vi "RunSelfCheck5.vi"(1 "Select_CalPwrMeters":bool=TRUE, 2 "Select_SplitterPwr":bool=TRUE, 3 "error in (no error)":errorcluster, 4 "Select_Processor_HV_Flag":bool=TRUE, 5 "File name base":string="SelfCheck5_") -> (0 "error out":errorcluster)   [LabVIEW 2009]
doc: "Measures a collection of system calibration variables, growing awith time, a work in progress."
uses:
  Rvp8PowerData.ctl
panel:
  in  "startGateTestPulse":i32=970
  in  "nGates TestPulse":i32=10
  in  "nSamplesTestPulse":i32=1000
  out "RVP8_testPulse_measurement":T1 {"time" format="%<%H:%M:%S\n%Y/%m/%d>T"}
  in  "SG Freq GHz 2":dbl=2.795 format="%#.5f"
  out "SelfCheckEndTime":timestamp
  out "SelfCheckStartTime":timestamp
  out "OutputFileName":string
  out "or Tee, Confirm That Pol Sw 7222 = 0 = SCPI closed = local control Tee, Confirm That Pol Sw 7222 = 1 = SCPI open for processor 2":i32
  out "For Tee, Confirm That Pol Sw 7223 = 0 =  SCPI closed \"honly\" 2":i32
  out "or Tee, Confirm That Pol Sw 7222 = 0 = SCPI closed = local control Tee, Confirm That Pol Sw 7222 = 1 = SCPI open for processor":i32
  out "For Tee, Confirm That Pol Sw 7223 = 0 =  SCPI closed \"honly\"":i32
  out "RVP8_Noise_Injection_NoAmp_Normal":T1 {"time" format="%<%H:%M:%S\n%Y/%m/%d>T"}
  out "RVP8_SigGen_NoAmp_Normal":T1 {"time" format="%<%H:%M:%S\n%Y/%m/%d>T"}
  out "dBAvg Power Meter Noise Floor (dBm)":dbl format="%#.5f"
  in  "startGate burst RVP8":i32=-1
  in  "nGates burst RVP8":i32=1
  in  "nSamples burst RVP8":i32=1000
  out "RVP8 TxBurstHc":dbl
  out "RVP8_burstPulse_measurement":T1 {"time" format="%<%H:%M:%S\n%Y/%m/%d>T"}
  out "String_WgSw_Positions":string
  out "Initial Check  of Transmit Detector: TxUp=0 if not transmitting":i32
  out "RVP8_HighSigGen_Injection_Reversed":T1 {"time" format="%<%H:%M:%S\n%Y/%m/%d>T"}
  out "RVP8_HighSigGen_Injection_Normal":T1 {"time" format="%<%H:%M:%S\n%Y/%m/%d>T"}
  out "Updating Data File Time":string
  out "StringOfRelayCycles":string
  out "SSD TOF Tx Pwr Reading dB":dbl format="%#.6g"
  out "TOF Tx Pwr Reading dBm":dbl format="%#.6g"
  out "dB SSD SigGen Power NO Amp to splitter (dB)":dbl format="%.5f"
  out "dBAvg SigGen Power NO Amp to splitter (dBm)":dbl format="%.3f"
  out "dB SSD Inside Noise Box Power thru Amp to splitter (dB)":dbl format="%.5f"
  out "dBSSD SigGen Power thru Amp to splitter (dB)":dbl format="%.5f"
  out "RVP8_LowSigGen_Injection_Normal":T1 {"time" format="%<%H:%M:%S\n%Y/%m/%d>T"}
  out "RVP8_LowSigGen_Injection_Reversed":T1 {"time" format="%<%H:%M:%S\n%Y/%m/%d>T"}
  out "StartFracDaysSince01Jan1904":dbl format="%#.6g"
  in  "File name exten":string="csv"
  out "TxDetector Voltage":dbl
  out "Temp Inside Noise Box":dbl
  out "Temp Outside Noise Box":dbl
  out "RVP8_Noise_Injection_Reversed":T1 {"time" format="%<%H:%M:%S\n%Y/%m/%d>T"}
  out "RVP8_Noise_Injection_Normal":T1 {"time" format="%<%H:%M:%S\n%Y/%m/%d>T"}
  out "RVP8_outside_noise_box_normal":T1 {"time" format="%<%H:%M:%S\n%Y/%m/%d>T"}
  out "First RVP8 Time":dbl format="%#_9g"
  out "RVP8_background_noise_normal":T1 {"time" format="%<%H:%M:%S\n%Y/%m/%d>T"}
  out "+15V PS Voltage":dbl
  out "+24V PS Voltage":dbl
  out "Temp 34921T":dbl
  out "Temp TOF Pwr Sensor":dbl
  out "Temp Klystron":dbl
  out "Temp DL V":dbl
  out "Temp DL H":dbl
  out "Temp Circ V":dbl
  out "Temp Circ H":dbl
  out "Temp Outside":dbl
  out "Temp Delay":dbl
  out "dBAvg Inside Noise Box Power Thru Amp to splitter (dBm)":dbl format="%.3f"
  out "Temp Amp":dbl
  out "Temp Inside":dbl
  out "Temp Siggen":dbl
  out "Temp IFD":dbl
  out "First RVP8 azimuth":dbl
  out "First RVP8 elevation":dbl
  out "Temp LNA  V":dbl
  out "Temp LNA H":dbl
  out "Temp Pwr Sensor":dbl
  out "dBAvg SigGen Power thru Amp to splitter (dBm)":dbl format="%.3f"
  in  "Cal data directory":string="/home/operator/data"
  # "RECEIVER AND TEST EQUIPMENT SELF CHECKS & LOGGING VERSION #5:"
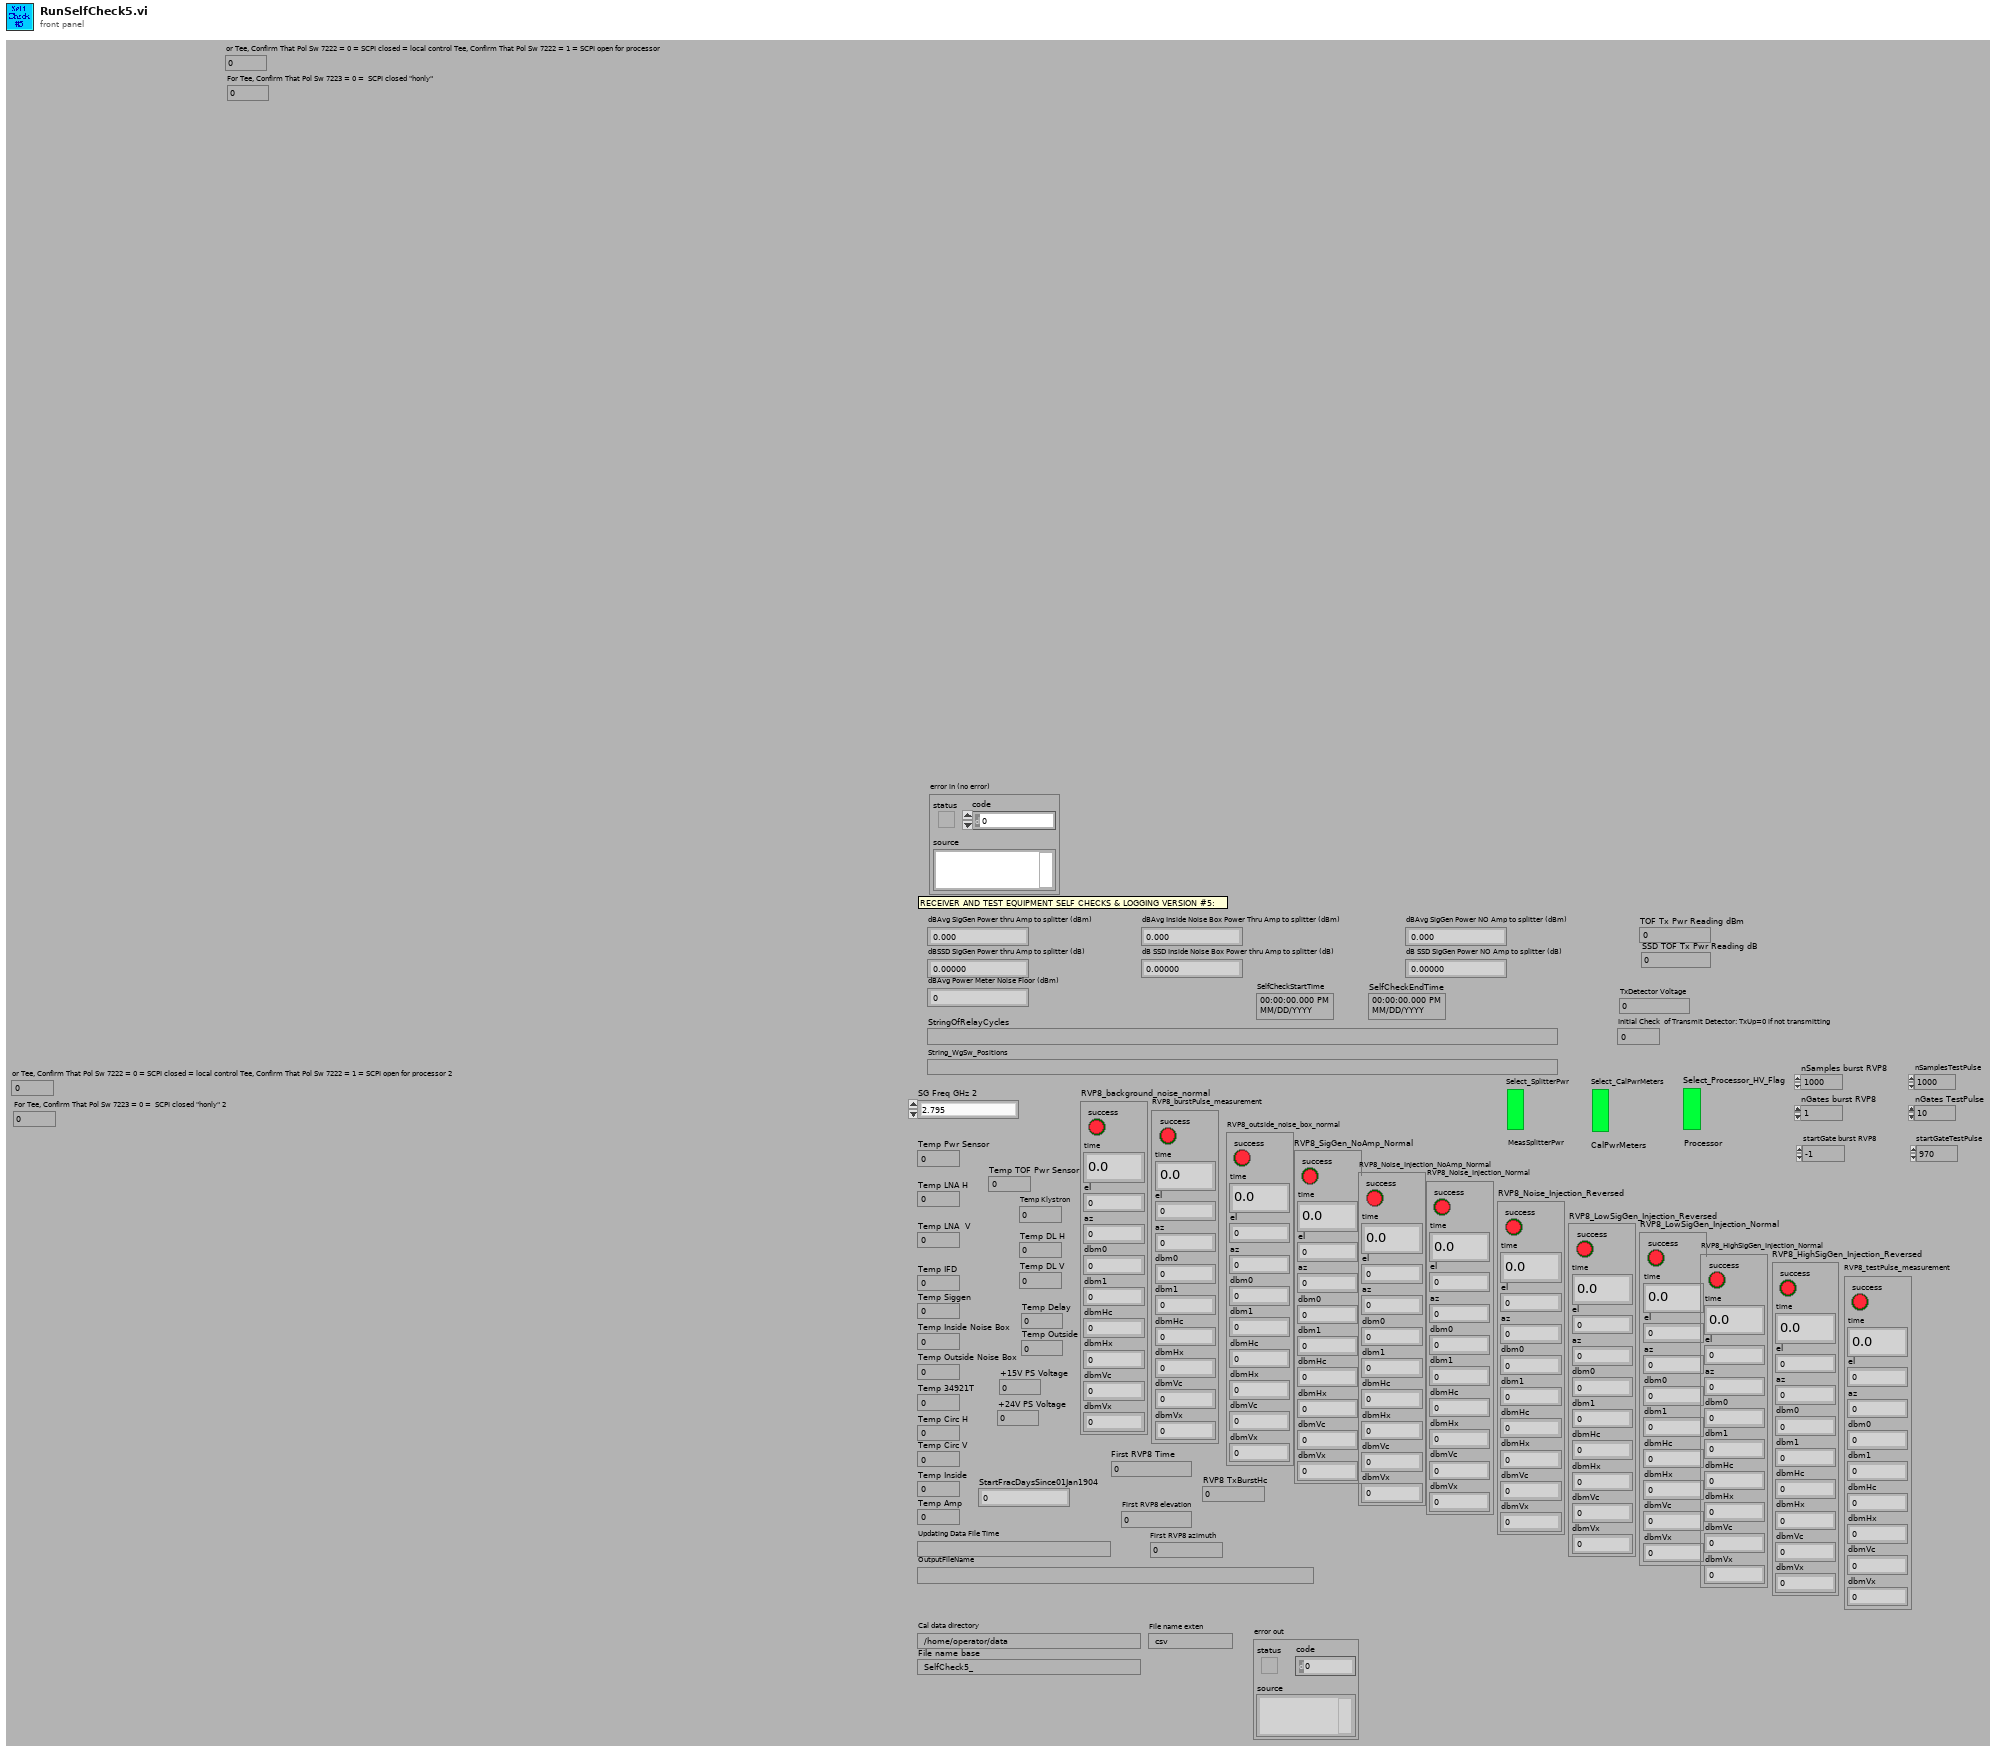
[diagram p1: front panel]
types:
  T1 = typedef "Rvp8PowerData.ctl" = cluster{"success":bool, "time":dbl, "el":dbl, "az":dbl, "dbm0":dbl, "dbm1":dbl, "dbmHc":dbl, "dbmHx":dbl, "dbmVc":dbl, "dbmVx":dbl}
  T2 = enum16{"open", "replace", "create", "open or create", "replace or create", "replace or create with confirmation"}
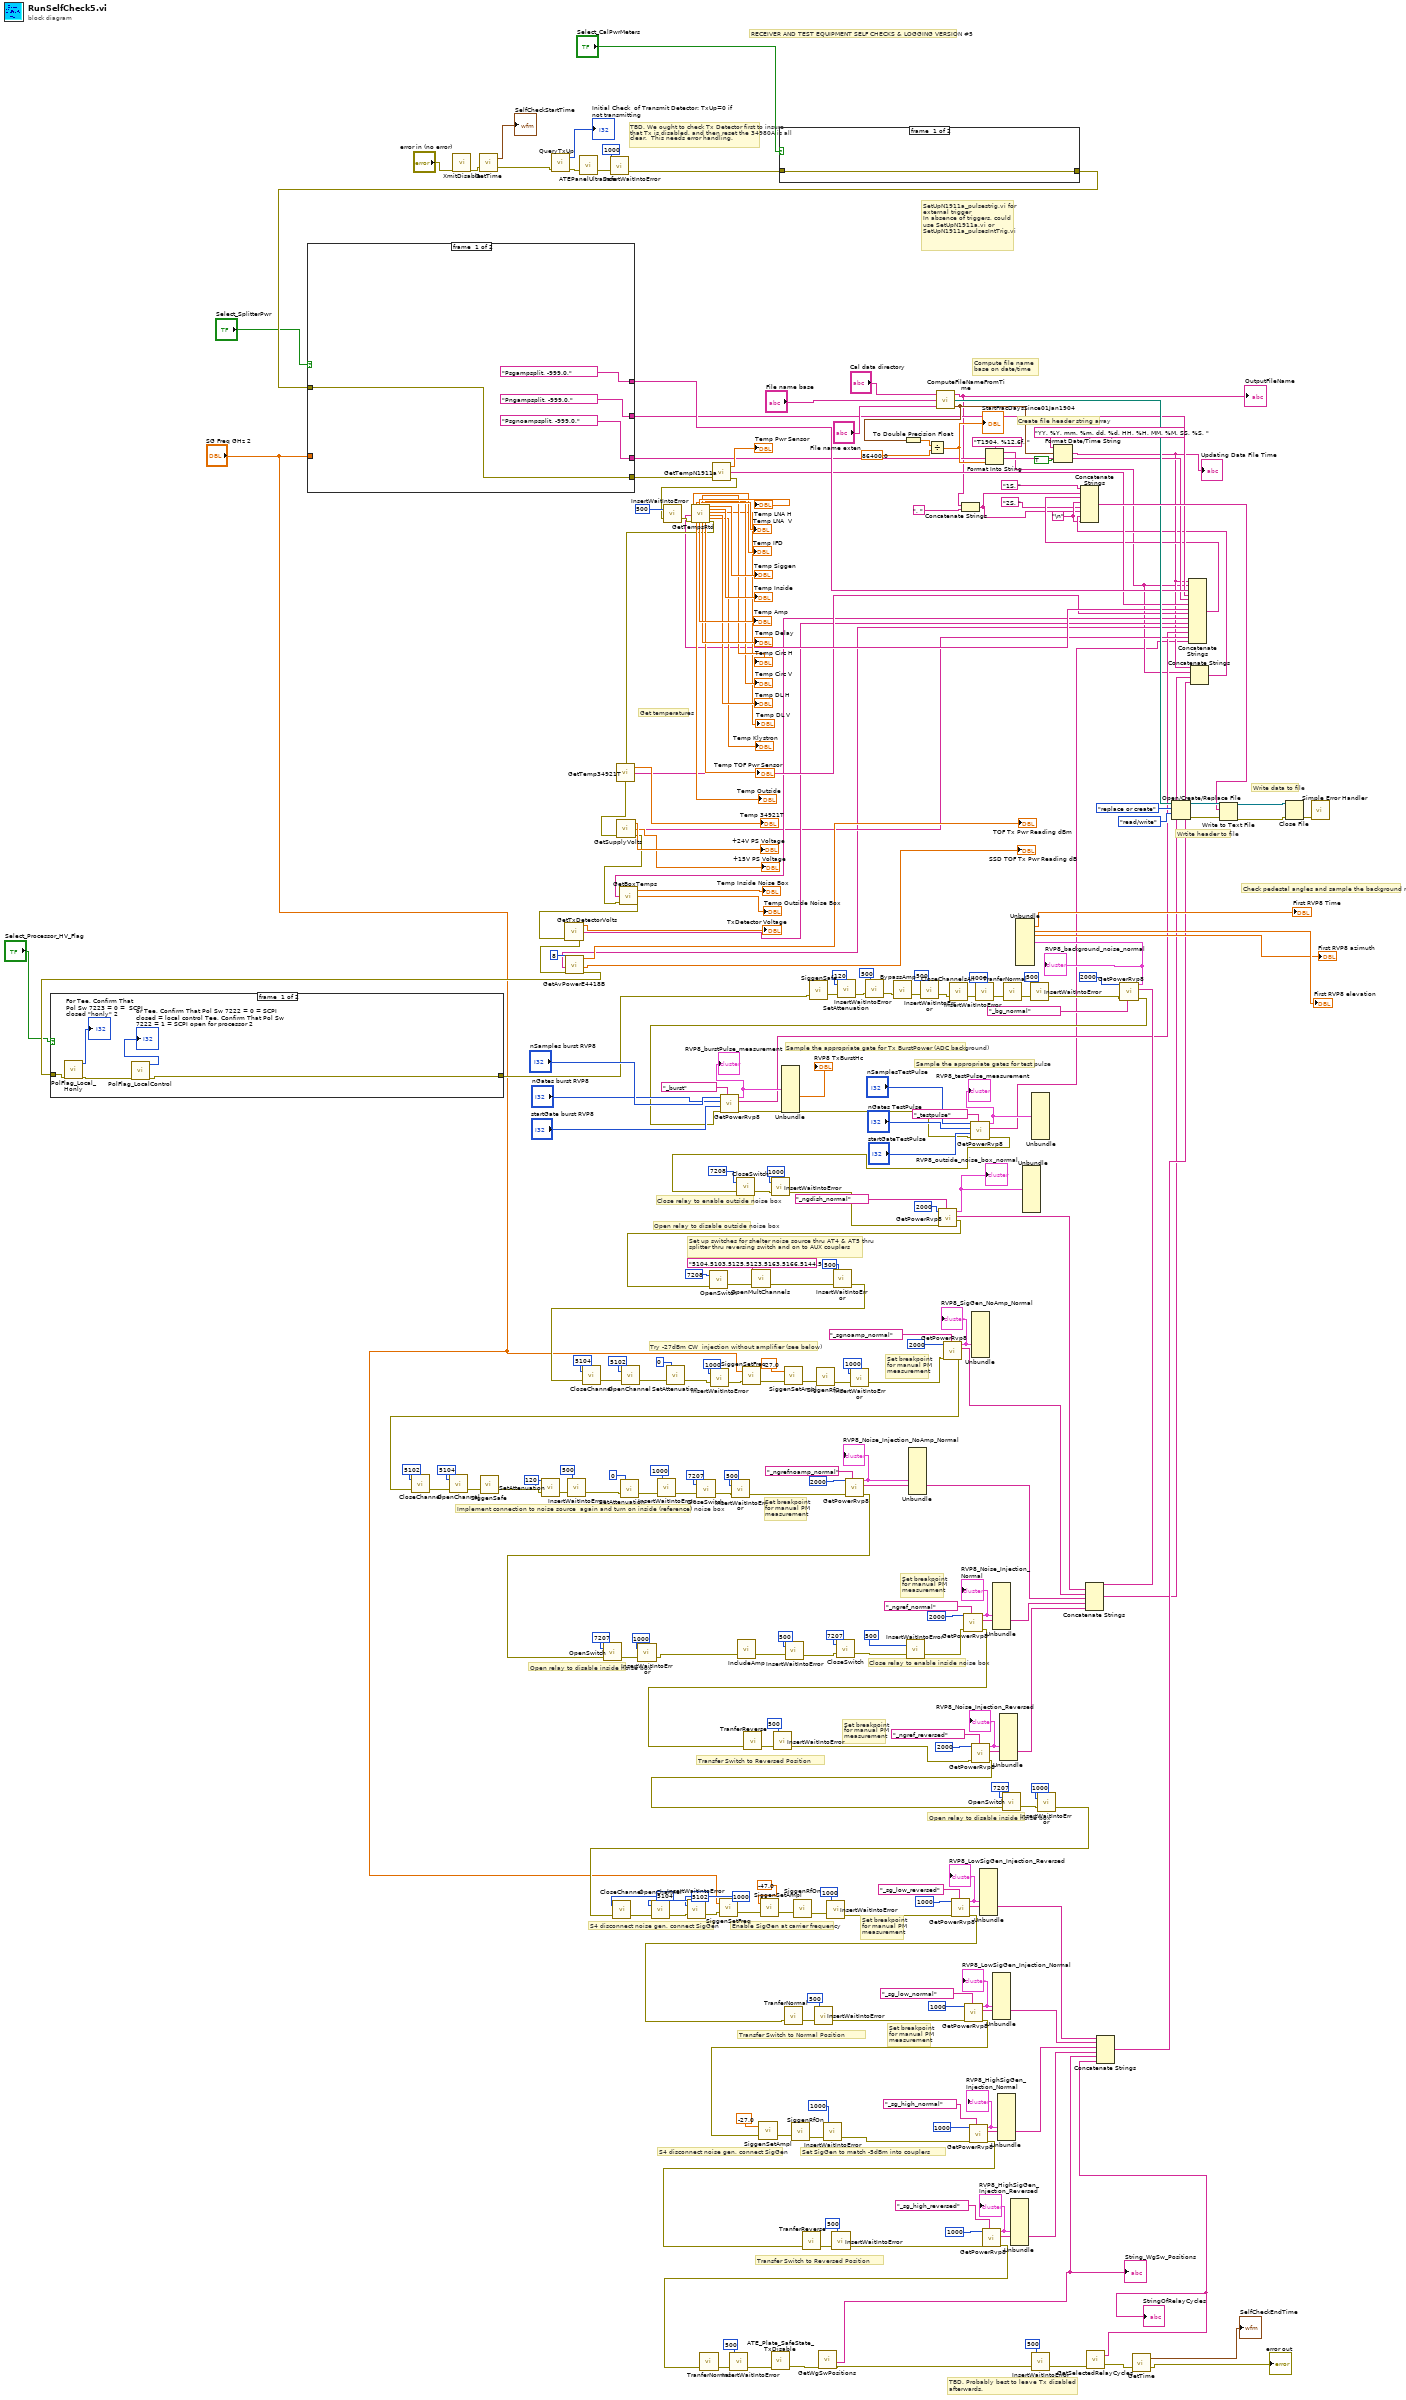
[diagram p0: block diagram]
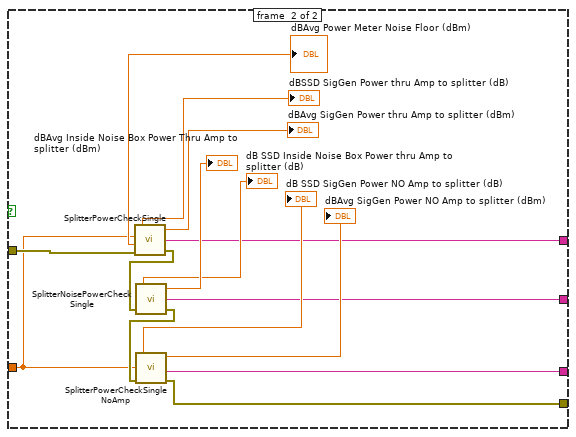
[diagram p2: hidden frame]
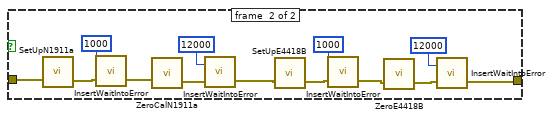
[diagram p3: hidden frame]
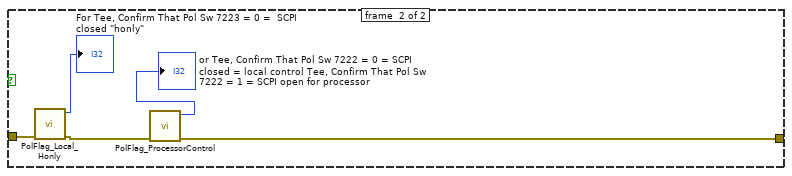
[diagram p4: hidden frame]
diagram:
  w80 = "\n"
  # "Sample the appropriate gates for test pulse"
  # "Set breakpoint for manual PM measurement"
  # "Set breakpoint for manual PM measurement"
  # "Set breakpoint for manual PM measurement"
  # "Set breakpoint for manual PM measurement"
  # "Set breakpoint for manual PM measurement"
  # "Set breakpoint for manual PM measurement"
  # "Open relay to disable inside noise box"
  # "Try -27dBm CW  injection without amplifier (see below)"
  # "Implement connection to noise source  again and turn on inside (reference) noise box"
  # "SetUpN1911a_pulsestrig.vi for external trigger\nIn absence of triggers, could use SetUpN1911a.vi or SetUpN1911a_pulsesIntTrig.vi"
  # "Sample the appropriate gate for Tx BurstPower (ADC background)"
  # "S4 disconnect noise gen, connect SigGen"
  # "Set SigGen to match -5dBm into couplers"
  # "Transfer Switch to Reversed Position"
  # "TBD. Probably best to leave Tx disabled afterwards."
  # "TBD. We ought to check Tx Detector first to insure that Tx is disabled, and then reset the 34980A is all clear.  This needs error handling."
  # "S4 disconnect noise gen, connect SigGen"
  # "Enable SigGen at carrier frequency"
  # "Transfer Switch to Normal Position"
  # "Transfer Switch to Reversed Position"
  # "Open relay to disable inside noise box"
  # "RECEIVER AND TEST EQUIPMENT SELF CHECKS & LOGGING VERSION #5"
  # "Close relay to enable inside noise box"
  # "Open relay to disable outside noise box"
  # "Close relay to enable outside noise box"
  # "Check pedestal angles and sample the background noise"
  # "Get temperatures"
  # "Write data to file"
  # "Wrtite header to file"
  # "Create file header string array"
  # "Set up switches for shelter noise source thru AT4 & AT5 thru splitter thru reversing switch and on to AUX couplers"
  # "Compute file name base on date/time"
  n1 = call "XmitDisable.vi"("error in (no error)"="error in (no error)") -> ("error out"=w15:errorcluster)  [unwired: 1 in, 5 out]
  n2 = call "GetTime.vi"("error in (no error)"=w15) -> ("error out"=w14:errorcluster, "CurrentTime"=→"SelfCheckStartTime":timestamp)  [unwired: 1 in]
  n3 = call "QueryTxUp.vi"("error in (no error)"=w14) -> ("error out"=w133:errorcluster, "IfTransmittingOne"=→"Initial Check  of Transmit Detector: TxUp=0 if not transmitting":i32)  [unwired: 1 in, 2 out]
  n4 = call "ATEPanelUltraSafe.vi"("error in (no error)"=w133) -> ("Error out"=w97:errorcluster)  [unwired: 2 in]
  n5 = call "InsertWaitIntoError.vi"("error in (no error)"=w97, "Wait (msecs)"=1000) -> ("error out"=w189:errorcluster)  [unwired: 1 in]
  n6 = case shown="True" "Select_CalPwrMeters" {
    tunnel: w189 -> [w267 w275]
    tunnel: [w267 w268] -> w154
    frame #0 {
    }
    frame #1 {
      n7 = call "SetUpN1911a.vi"("error in (no error)"=w275) -> ("error out"=w278:errorcluster)  [unwired: 2 in]
      n8 = call "InsertWaitIntoError.vi"("error in (no error)"=w278, "Wait (msecs)"=1000) -> ("error out"=w277:errorcluster)  [unwired: 1 in]
      n9 = call "ZeroCalN1911a.vi"("error in (no error)"=w277) -> ("error out"=w276:errorcluster)  [unwired: 2 in]
      n10 = call "InsertWaitIntoError.vi"("error in (no error)"=w276, "Wait (msecs)"=12000) -> ("error out"=w269:errorcluster)  [unwired: 1 in]
      n11 = call "SetUpE4418B.vi"("error in (no error)"=w269) -> ("error out"=w272:errorcluster)  [unwired: 2 in]
      n12 = call "InsertWaitIntoError.vi"("error in (no error)"=w272, "Wait (msecs)"=1000) -> ("error out"=w271:errorcluster)  [unwired: 1 in]
      n13 = call "ZeroE4418B.vi"("error in (no error)"=w271) -> ("error out"=w270:errorcluster)  [unwired: 2 in]
      n14 = call "InsertWaitIntoError.vi"("error in (no error)"=w270, "Wait (msecs)"=12000) -> ("error out"=w268:errorcluster)  [unwired: 1 in]
    }
  }
  n15 = case shown="True" "Select_SplitterPwr" {
    tunnel: [w284 w296] -> w155
    tunnel: w154 -> [w284 w290]
    tunnel: ["Psgampsplit, -999.0," w289] -> w118
    tunnel: ["Pngampsplit, -999.0," w288] -> w117
    tunnel: ["Psgnoampsplit, -999.0," w287] -> w116
    tunnel: "SG Freq GHz 2" -> [_ w285]
    frame #0 {
    }
    frame #1 {
      n16 = call "SplitterPowerCheckSingle.vi"("error in (no error)"=w290, "Select SG Freq GHz"=w285) -> ("error out"=w298:errorcluster, "String_PSG_Amp_Split"=w289:string, "dBAvg SigGen Power to splitter (dBm)"=→"dBAvg SigGen Power thru Amp to splitter (dBm)":dbl, "dBAvg Power Meter Noise Floor (dBm)"=→"dBAvg Power Meter Noise Floor (dBm)":dbl, "dBSSD SigGen Power to splitter (dB)"=→"dBSSD SigGen Power thru Amp to splitter (dB)":dbl)
      n17 = call "SplitterNoisePowerCheckSingle.vi"("error in (no error)"=w298) -> ("error out"=w295:errorcluster, "String_PNG_Amp_Split"=w288:string, "dBAvg Noise Power to splitter (dBm)"=→"dBAvg Inside Noise Box Power Thru Amp to splitter (dBm)":dbl, "dBSSD Noise Power to splitter (dB)"=→"dB SSD Inside Noise Box Power thru Amp to splitter (dB)":dbl)  [unwired: 1 in]
      n18 = call "SplitterPowerCheckSingleNoAmp.vi"("error in (no error)"=w295, "Select SG Freq GHz"=w285) -> ("error out"=w296:errorcluster, "String_PSG_Noamp_Split"=w287:string, "dBAvg SigGen Power to splitter (dBm)"=→"dBAvg SigGen Power NO Amp to splitter (dBm)":dbl, "dBSSD SigGen Power to splitter (dB)"=→"dB SSD SigGen Power NO Amp to splitter (dB)":dbl)  [unwired: 1 in, 1 out]
    }
  }
  n19 = call "GetTempN1911a.vi"("error in (no error)"=w155) -> ("Error out"=w250:errorcluster, "String_Temp_n1911a"=w115:string, "N1911a Temp (C)"=→"Temp Pwr Sensor":dbl)  [unwired: 2 in]
  n20 = call "InsertWaitIntoError.vi"("error in (no error)"=w250, "Wait (msecs)"=500) -> ("error out"=w252:errorcluster)  [unwired: 1 in]
  n21 = call "GetTempsRtd.vi"("error in (no error)"=w252) -> ("Temp IFD"=→"Temp IFD":dbl, "String_Temperatures"=w114:string, "Temp VLNA"=→"Temp LNA  V":dbl, "Temp Outside"=→"Temp Outside":dbl, "Temp HLNA"=→"Temp LNA H":dbl, "Temp ATE Amp"=→"Temp Amp":dbl, "Temp H Circ"=→"Temp Circ H":dbl, "Temp ATE delay"=→"Temp Delay":dbl, "Temp V Circ"=→"Temp Circ V":dbl, "Temp TOF Pwr"=→"Temp TOF Pwr Sensor":dbl, "Temp Siggen"=→"Temp Siggen":dbl, "Temp Inside"=→"Temp Inside":dbl, "Temp V Dummy"=→"Temp DL V":dbl, "Temp H Dummy"=→"Temp DL H":dbl, "Temp Klystron"=→"Temp Klystron":dbl, "error out"=w232:errorcluster)  [unwired: 2 in, 1 out]
  n22 = call "GetTemp34921T.vi"("error in (no error)"=w232) -> ("Error out"=w233:errorcluster, "String_Temp_34921T"=w113:string, "34921A Temp (C)"=→"Temp 34921T":dbl)  [unwired: 2 in]
  n23 = call "GetSupplyVolts.vi"("error in (no error)"=w233) -> ("error out"=w197:errorcluster, "String_Volts"=w99:string, "Volts +15"=→"+15V PS Voltage":dbl, "Volts +24"=→"+24V PS Voltage":dbl)  [unwired: 1 in]
  n24 = call "GetBoxTemps.vi"("error in (no error)"=w197) -> ("error out"=w196:errorcluster, "Outside Box"=→"Temp Outside Noise Box":dbl, "InsideBox"=→"Temp Inside Noise Box":dbl, "String_Temp_NoiseBoxes"=w112:string)  [unwired: 1 in]
  n25 = call "GetTxDetectorVolts.vi"("error in (no error)"=w196) -> ("error out"=w152:errorcluster, "String_Volts_TxDet"=w111:string, "Volts Tx Detector"=→"TxDetector Voltage":dbl)  [unwired: 2 in]
  n26 = call "GetAvPowerE4418B.vi"("error in (no error)"=w152, "N samples"=8) -> ("Error out"=w23:errorcluster, "VI dBSSD Power (dB)"=→"SSD TOF Tx Pwr Reading dB":dbl, "VI Mean Power (dBm)"=→"TOF Tx Pwr Reading dBm":dbl, "String_E4418A_Pwr"=w95:string)  [unwired: 2 in]
  n27 = case shown="True" "Select_Processor_HV_Flag" {
    tunnel: w23 -> [w301 w306]
    tunnel: [w300 w305] -> w22
    frame #0 {
      n28 = call "PolFlag_Local_Honly.vi"("error in (no error)"=w301) -> ("error out"=w303:errorcluster, "Position (0=open, 1=closed)"=→"For Tee, Confirm That Pol Sw 7223 = 0 =  SCPI closed \"honly\" 2":i32)  [unwired: 3 in, 2 out]
      n29 = call "PolFlag_LocalControl.vi"("error in (no error)"=w303) -> ("error out"=w300:errorcluster, "Position (0=open, 1=closed)"=→"or Tee, Confirm That Pol Sw 7222 = 0 = SCPI closed = local control Tee, Confirm That Pol Sw 7222 = 1 = SCPI open for processor 2":i32)  [unwired: 3 in, 2 out]
    }
    frame #1 {
      n30 = call "PolFlag_Local_Honly.vi"("error in (no error)"=w306) -> ("error out"=w308:errorcluster, "Position (0=open, 1=closed)"=→"For Tee, Confirm That Pol Sw 7223 = 0 =  SCPI closed \"honly\"":i32)  [unwired: 3 in, 2 out]
      n31 = call "PolFlag_ProcessorControl.vi"("error in (no error)"=w308) -> ("error out"=w305:errorcluster, "Position (0=open, 1=closed)"=→"or Tee, Confirm That Pol Sw 7222 = 0 = SCPI closed = local control Tee, Confirm That Pol Sw 7222 = 1 = SCPI open for processor":i32)  [unwired: 3 in, 2 out]
    }
  }
  n32 = call "SiggenSafe.vi"("error in (no error)"=w22) -> ("error out"=w214:errorcluster)  [unwired: 2 in]
  n33 = call "SetAttenuation.vi"("error in (no error)"=w214, "Attenuation (dB)"=120) -> ("error out"=w212:errorcluster)  [unwired: 1 in]
  n34 = call "InsertWaitIntoError.vi"("error in (no error)"=w212, "Wait (msecs)"=500) -> ("error out"=w211:errorcluster)  [unwired: 1 in]
  n35 = call "BypassAmp.vi"("error in (no error)"=w211) -> ("error out"=w187:errorcluster)  [unwired: 2 in]
  n36 = call "InsertWaitIntoError.vi"("error in (no error)"=w187, "Wait (msecs)"=500) -> ("error out"=w186:errorcluster)  [unwired: 1 in]
  n37 = call "ComputeFileNameFromTime.vi"("File name extension"="File name exten", "File name base"="File name base", "Output directory"="Cal data directory") -> ("TIme used"=w177:timestamp, "Output file path"=w254:path, "Output file name"=w19:string)
  "OutputFileName" <- w19
  n38 = To Double Precision Float(number=w177) -> (double precision float=w176:dbl)
  n39 = Divide(x=w176, y=86400.0) -> (x/y=w119:dbl)
  "StartFracDaysSince01Jan1904" <- w119
  n40 = call "CloseChannelsAll.vi"("error in (no error)"=w186) -> ("error out"=w264:errorcluster)  [unwired: 2 in]
  n41 = Concatenate Strings(w19, ", ") -> (w18:string)
  n42 = call "InsertWaitIntoError.vi"("error in (no error)"=w264, "Wait (msecs)"=4000) -> ("error out"=w199:errorcluster)  [unwired: 1 in]
  n43 = Format Into String(format string="T1904, %12.6f, ", w119) -> (resulting string=w82:string)  [unwired: 2 in, 1 out]
  n44 = call "TranferNormal.vi"("error in (no error)"=w199) -> ("error out"=w184:errorcluster)  [unwired: 2 in]
  n45 = call "InsertWaitIntoError.vi"("error in (no error)"=w184, "Wait (msecs)"=500) -> ("error out"=w183:errorcluster)  [unwired: 1 in]
  n46 = Format Date/Time String(time format string (%c)="YY, %Y, mm, %m, dd, %d, HH, %H, MM, %M, SS, %S, ", seconds (now)=w177, UTC format=TRUE) -> (date/time string=w85:string)
  "Updating Data File Time" <- w85
  n47 = call "GetPowerRvp8.vi"("SpecifyTypeOfDataAcq"="_bg_normal", "error in (no error)"=w183, "nSamples"=2000) -> ("Comm error"=w87:errorcluster, "String_of_RVP8_Powers"=w106:string, "RVP8_power"=w227:T1)  [unwired: 2 in, 1 out]
  "RVP8_background_noise_normal" <- w227
  n48 = call "GetPowerRvp8.vi"("SpecifyTypeOfDataAcq"="_burst", "error in (no error)"=w87, "startGate"="startGate burst RVP8", "nGates"="nGates burst RVP8", "nSamples"="nSamples burst RVP8") -> ("Comm error"=w3:errorcluster, "String_of_RVP8_Powers"=w88:string, "RVP8_power"=w94:T1)  [unwired: 1 out]
  "RVP8_burstPulse_measurement" <- w94
  n49 = Unbundle(w94) -> ("dbmHc"=→"RVP8 TxBurstHc":dbl)  [unwired: 9 out]
  n50 = call "GetPowerRvp8.vi"("SpecifyTypeOfDataAcq"="_testpulse", "error in (no error)"=w3, "startGate"="startGateTestPulse", "nGates"="nGates TestPulse", "nSamples"="nSamplesTestPulse") -> ("Comm error"=w2:errorcluster, "String_of_RVP8_Powers"=w1:string, "RVP8_power"=w8:T1)  [unwired: 1 out]
  "RVP8_testPulse_measurement" <- w8
  n51 = call "CloseSwitch.vi"("error in (no error)"=w2, "Switch ID"=7208) -> ("error out"=w224:errorcluster)  [unwired: 1 in]
  n52 = call "InsertWaitIntoError.vi"("error in (no error)"=w224, "Wait (msecs)"=1000) -> ("error out"=w220:errorcluster)  [unwired: 1 in]
  n53 = call "GetPowerRvp8.vi"("SpecifyTypeOfDataAcq"="_ngdish_normal", "error in (no error)"=w220, "nSamples"=2000) -> ("XML error"=w218:errorcluster, "String_of_RVP8_Powers"=w105:string, "RVP8_power"=w222:T1)  [unwired: 2 in, 1 out]
  "RVP8_outside_noise_box_normal" <- w222
  n54 = call "OpenSwitch.vi"("error in (no error)"=w218, "Switch ID"=7208) -> ("error out"=w217:errorcluster)  [unwired: 1 in]
  n55 = call "OpenMultChannels.vi"("error in (no error)"=w217, "Channels to be opened"="5104,5103,5125,5123,5163,5166,5144,5141") -> ("error out"=w181:errorcluster)  [unwired: 1 in]
  n56 = call "InsertWaitIntoError.vi"("error in (no error)"=w181, "Wait (msecs)"=500) -> ("error out"=w61:errorcluster)  [unwired: 1 in]
  n57 = call "CloseChannel.vi"("error in (no error)"=w61, "Channel ID"=5104) -> ("error out"=w66:errorcluster)  [unwired: 1 in]
  n58 = call "OpenChannel.vi"("error in (no error)"=w66, "Channel ID"=5102) -> ("error out"=w64:errorcluster)  [unwired: 1 in]
  n59 = call "SetAttenuation.vi"("error in (no error)"=w64, "Attenuation (dB)"=0) -> ("error out"=w63:errorcluster)  [unwired: 1 in]
  n60 = call "InsertWaitIntoError.vi"("error in (no error)"=w63, "Wait (msecs)"=1000) -> ("error out"=w65:errorcluster)  [unwired: 1 in]
  n61 = call "SiggenSetFreq.vi"("error in (no error)"=w65, "Freq request (GHz)"="SG Freq GHz 2") -> ("Error status"=w72:errorcluster)  [unwired: 1 out]
  n62 = call "SiggenSetAmpl.vi"("error in (no error)"=w72, "Amplitude request (dBm)"=-27.0) -> ("error out"=w70:errorcluster)  [unwired: 1 out]
  n63 = call "SiggenRfOn.vi"("error in (no error)"=w70) -> ("error out"=w62:errorcluster)  [unwired: 2 in]
  n64 = call "InsertWaitIntoError.vi"("error in (no error)"=w62, "Wait (msecs)"=1000) -> ("error out"=w75:errorcluster)  [unwired: 1 in]
  n65 = call "GetPowerRvp8.vi"("SpecifyTypeOfDataAcq"="_sgnoamp_normal", "error in (no error)"=w75, "nSamples"=2000) -> ("Comm error"=w57:errorcluster, "String_of_RVP8_Powers"=w56:string, "RVP8_power"=w77:T1)  [unwired: 2 in, 1 out]
  "RVP8_SigGen_NoAmp_Normal" <- w77
  n66 = call "CloseChannel.vi"("error in (no error)"=w57, "Channel ID"=5102) -> ("error out"=w58:errorcluster)  [unwired: 1 in]
  n67 = call "OpenChannel.vi"("error in (no error)"=w58, "Channel ID"=5104) -> ("error out"=w44:errorcluster)  [unwired: 1 in]
  n68 = call "SiggenSafe.vi"("error in (no error)"=w44) -> ("error out"=w54:errorcluster)  [unwired: 2 in]
  n69 = call "SetAttenuation.vi"("error in (no error)"=w54, "Attenuation (dB)"=120) -> ("error out"=w48:errorcluster)  [unwired: 1 in]
  n70 = call "InsertWaitIntoError.vi"("error in (no error)"=w48, "Wait (msecs)"=500) -> ("error out"=w43:errorcluster)  [unwired: 1 in]
  n71 = call "SetAttenuation.vi"("error in (no error)"=w43, "Attenuation (dB)"=0) -> ("error out"=w46:errorcluster)  [unwired: 1 in]
  n72 = call "InsertWaitIntoError.vi"("error in (no error)"=w46, "Wait (msecs)"=1000) -> ("error out"=w45:errorcluster)  [unwired: 1 in]
  n73 = call "CloseSwitch.vi"("error in (no error)"=w45, "Switch ID"=7207) -> ("error out"=w51:errorcluster)  [unwired: 1 in]
  n74 = call "InsertWaitIntoError.vi"("error in (no error)"=w51, "Wait (msecs)"=500) -> ("error out"=w39:errorcluster)  [unwired: 1 in]
  n75 = call "GetPowerRvp8.vi"("SpecifyTypeOfDataAcq"="_ngrefnoamp_normal", "error in (no error)"=w39, "nSamples"=2000) -> ("Comm error"=w35:errorcluster, "String_of_RVP8_Powers"=w30:string, "RVP8_power"=w41:T1)  [unwired: 2 in, 1 out]
  "RVP8_Noise_Injection_NoAmp_Normal" <- w41
  n76 = call "OpenSwitch.vi"("error in (no error)"=w35, "Switch ID"=7207) -> ("error out"=w36:errorcluster)  [unwired: 1 in]
  n77 = call "InsertWaitIntoError.vi"("error in (no error)"=w36, "Wait (msecs)"=1000) -> ("error out"=w34:errorcluster)  [unwired: 1 in]
  n78 = call "IncludeAmp.vi"("error in (no error)"=w34) -> ("error out"=w32:errorcluster)  [unwired: 2 in]
  n79 = call "InsertWaitIntoError.vi"("error in (no error)"=w32, "Wait (msecs)"=500) -> ("error out"=w31:errorcluster)  [unwired: 1 in]
  n80 = call "CloseSwitch.vi"("error in (no error)"=w31, "Switch ID"=7207) -> ("error out"=w208:errorcluster)  [unwired: 1 in]
  n81 = call "InsertWaitIntoError.vi"("error in (no error)"=w208, "Wait (msecs)"=500) -> ("error out"=w207:errorcluster)  [unwired: 1 in]
  n82 = Unbundle(w41) -> ()  [unwired: 10 out]
  n83 = call "GetPowerRvp8.vi"("SpecifyTypeOfDataAcq"="_ngref_normal", "error in (no error)"=w207, "nSamples"=2000) -> ("Comm error"=w198:errorcluster, "String_of_RVP8_Powers"=w104:string, "RVP8_power"=w216:T1)  [unwired: 2 in, 1 out]
  "RVP8_Noise_Injection_Normal" <- w216
  n84 = call "TranferReverse.vi"("error in (no error)"=w198) -> ("error out"=w179:errorcluster)  [unwired: 2 in]
  n85 = call "InsertWaitIntoError.vi"("error in (no error)"=w179, "Wait (msecs)"=500) -> ("error out"=w178:errorcluster)  [unwired: 1 in]
  n86 = Unbundle(w77) -> ()  [unwired: 10 out]
  n87 = call "GetPowerRvp8.vi"("SpecifyTypeOfDataAcq"="_ngref_reversed", "error in (no error)"=w178, "nSamples"=2000) -> ("Comm error"=w202:errorcluster, "String_of_RVP8_Powers"=w103:string, "RVP8_power"=w201:T1)  [unwired: 2 in, 1 out]
  "RVP8_Noise_Injection_Reversed" <- w201
  n88 = Unbundle(w216) -> ()  [unwired: 10 out]
  n89 = Unbundle(w201) -> ()  [unwired: 10 out]
  n90 = call "OpenSwitch.vi"("error in (no error)"=w202, "Switch ID"=7207) -> ("error out"=w203:errorcluster)  [unwired: 1 in]
  n91 = Unbundle(w227) -> ("time"=→"First RVP8 Time":dbl, "el"=→"First RVP8 elevation":dbl, "az"=→"First RVP8 azimuth":dbl)  [unwired: 7 out]
  n92 = Unbundle(w222) -> ()  [unwired: 10 out]
  n93 = Unbundle(w8) -> ()  [unwired: 10 out]
  n94 = call "InsertWaitIntoError.vi"("error in (no error)"=w203, "Wait (msecs)"=1000) -> ("error out"=w160:errorcluster)  [unwired: 1 in]
  n95 = call "CloseChannel.vi"("error in (no error)"=w160, "Channel ID"=5104) -> ("error out"=w159:errorcluster)  [unwired: 1 in]
  n96 = call "OpenChannel.vi"("error in (no error)"=w159, "Channel ID"=5102) -> ("error out"=w158:errorcluster)  [unwired: 1 in]
  n97 = call "InsertWaitIntoError.vi"("error in (no error)"=w158, "Wait (msecs)"=1000) -> ("error out"=w157:errorcluster)  [unwired: 1 in]
  n98 = call "SiggenSetFreq.vi"("error in (no error)"=w157, "Freq request (GHz)"="SG Freq GHz 2") -> ("Error status"=w172:errorcluster)  [unwired: 1 out]
  n99 = call "SiggenSetAmpl.vi"("error in (no error)"=w172, "Amplitude request (dBm)"=-47.0) -> ("error out"=w164:errorcluster)  [unwired: 1 out]
  n100 = call "SiggenRfOn.vi"("error in (no error)"=w164) -> ("error out"=w28:errorcluster)  [unwired: 2 in]
  n101 = call "InsertWaitIntoError.vi"("error in (no error)"=w28, "Wait (msecs)"=1000) -> ("error out"=w27:errorcluster)  [unwired: 1 in]
  n102 = call "GetPowerRvp8.vi"("SpecifyTypeOfDataAcq"="_sg_low_reversed", "error in (no error)"=w27, "nSamples"=1000) -> ("Comm error"=w166:errorcluster, "String_of_RVP8_Powers"=w110:string, "RVP8_power"=w173:T1)  [unwired: 2 in, 1 out]
  "RVP8_LowSigGen_Injection_Reversed" <- w173
  n103 = call "TranferNormal.vi"("error in (no error)"=w166) -> ("error out"=w167:errorcluster)  [unwired: 2 in]
  n104 = call "InsertWaitIntoError.vi"("error in (no error)"=w167, "Wait (msecs)"=500) -> ("error out"=w165:errorcluster)  [unwired: 1 in]
  n105 = call "GetPowerRvp8.vi"("SpecifyTypeOfDataAcq"="_sg_low_normal", "error in (no error)"=w165, "nSamples"=1000) -> ("Comm error"=w138:errorcluster, "String_of_RVP8_Powers"=w109:string, "RVP8_power"=w169:T1)  [unwired: 2 in, 1 out]
  "RVP8_LowSigGen_Injection_Normal" <- w169
  n106 = call "SiggenSetAmpl.vi"("error in (no error)"=w138, "Amplitude request (dBm)"=-27.0) -> ("error out"=w139:errorcluster)  [unwired: 1 out]
  n107 = call "SiggenRfOn.vi"("error in (no error)"=w139) -> ("error out"=w26:errorcluster)  [unwired: 2 in]
  n108 = call "InsertWaitIntoError.vi"("error in (no error)"=w26, "Wait (msecs)"=1000) -> ("error out"=w25:errorcluster)  [unwired: 1 in]
  n109 = call "GetPowerRvp8.vi"("SpecifyTypeOfDataAcq"="_sg_high_normal", "error in (no error)"=w25, "nSamples"=1000) -> ("Comm error"=w141:errorcluster, "String_of_RVP8_Powers"=w108:string, "RVP8_power"=w147:T1)  [unwired: 2 in, 1 out]
  "RVP8_HighSigGen_Injection_Normal" <- w147
  n110 = call "TranferReverse.vi"("error in (no error)"=w141) -> ("error out"=w142:errorcluster)  [unwired: 2 in]
  n111 = call "InsertWaitIntoError.vi"("error in (no error)"=w142, "Wait (msecs)"=500) -> ("error out"=w140:errorcluster)  [unwired: 1 in]
  n112 = Unbundle(w173) -> ()  [unwired: 10 out]
  n113 = call "GetPowerRvp8.vi"("SpecifyTypeOfDataAcq"="_sg_high_reversed", "error in (no error)"=w140, "nSamples"=1000) -> ("Comm error"=w135:errorcluster, "String_of_RVP8_Powers"=w107:string, "RVP8_power"=w144:T1)  [unwired: 2 in, 1 out]
  "RVP8_HighSigGen_Injection_Reversed" <- w144
  n114 = call "TranferNormal.vi"("error in (no error)"=w135) -> ("error out"=w136:errorcluster)  [unwired: 2 in]
  n115 = call "InsertWaitIntoError.vi"("error in (no error)"=w136, "Wait (msecs)"=500) -> ("error out"=w134:errorcluster)  [unwired: 1 in]
  n116 = call "ATE_Plate_SafeState_TxDisable.vi"("error in (no error)"=w134) -> ("error out"=w121:errorcluster)  [unwired: 2 in]
  n117 = call "GetWgSwPositions.vi"("error in (no error)"=w121) -> ("error out"=w98:errorcluster, "String_WgSw_Positions"=w102:string)  [unwired: 5 out]
  "String_WgSw_Positions" <- w102
  n118 = Unbundle(w169) -> ()  [unwired: 10 out]
  n119 = Unbundle(w147) -> ()  [unwired: 10 out]
  n120 = Unbundle(w144) -> ()  [unwired: 10 out]
  n121 = call "InsertWaitIntoError.vi"("error in (no error)"=w98, "Wait (msecs)"=500) -> ("error out"=w149:errorcluster)  [unwired: 1 in]
  n122 = Concatenate Strings(w106, w105, w56, w30, w104, w103) -> (w84:string)
  n123 = call "GetSelectedRelayCycles.vi"("error in (no error)"=w149) -> ("error out"=w12:errorcluster, "StringOfRelayCycles"=w101:string)  [unwired: 1 in]
  "StringOfRelayCycles" <- w101
  n124 = Concatenate Strings(w110, w109, w108, w107, w102, w101) -> (w86:string)
  n125 = call "GetTime.vi"("error in (no error)"=w12) -> ("error out"=→"error out":errorcluster, "CurrentTime"=→"SelfCheckEndTime":timestamp)  [unwired: 1 in]
  n126 = Open/Create/Replace File(file path (use dialog)=w254, operation (0:open)=T2."replace or create", access (0:read/write)=enum16{"read/write", "read-only", "write-only"}."read/write") -> (refnum out=w260:refnum<file>, error out=w259:errorcluster)  [unwired: 3 in, 1 out]
  n127 = Concatenate Strings(w85, w82, w118, w117, w116, w115, w114, w113, w112, w111, w95, w88, w99, w1) -> (w100:string)
  n128 = Concatenate Strings(w85, w82, w84, w86) -> (w83:string)
  n129 = Concatenate Strings("1S, ", w18, w100, w80, "2S, ", w18, w83, w80) -> (w256:string)
  n130 = Write to Text File(file (use dialog)=w260, text=w256, error in=w259) -> (refnum out=w229:refnum<file>, error out=w228:errorcluster)  [unwired: 1 in, 1 out]
  n131 = Close File(refnum=w229, error in=w228) -> (error out=w261:errorcluster)  [unwired: 1 out]
  n132 = call <vilib>:"Simple Error Handler.vi"("error in (no error)"=w261) -> ()  [unwired: 4 in, 5 out]
